vi "Execute Commands.vi"(8 "error in (no error)":errorcluster, 10 "Command Array":refnum<class "Command.lvclass">[](array[class]), 11 "Command Handler in":refnum<class "Command Handler.lvclass">) -> (0 "error out":errorcluster, 3 "Command Handler out":refnum<class "Command Handler.lvclass">)   [LabVIEW 2015, in "Command Handler.lvlib" / "Command Handler.lvclass"]
uses:
  Command Handler.lvclass
  Command Handler Messages/Command Handler Global API/Command Handler Global.vi
  Command Handler.lvlib
  Command Parent/Command.lvclass
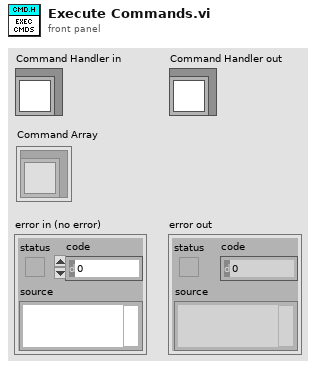
[diagram p1: front panel]
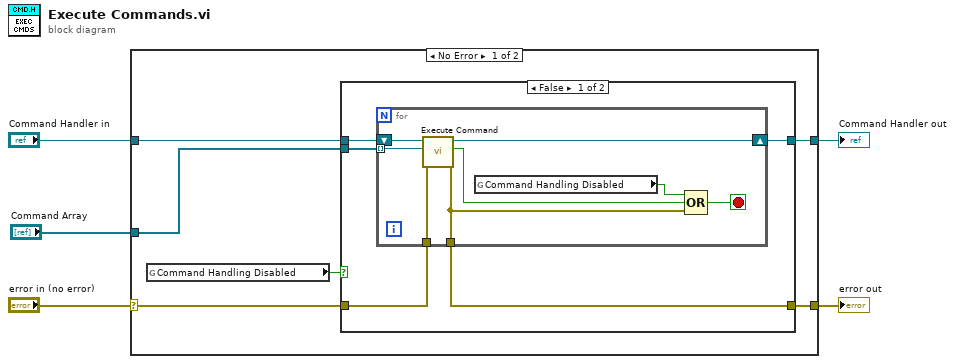
[diagram p0: block diagram]
diagram:
  n1 = case shown="No Error" "error in (no error)" {
    selector: "error in (no error)" -> [w10 w28]
    tunnel: [w9 w28] -> w4
    tunnel: [w7 w27] -> w2
    tunnel: "Command Handler in" -> [w8 w27]
    tunnel: "Command Array" -> [w11 _]
    frame No Error {
      n2 = global read "Command Handler Global.vi" "Command Handling Disabled"() -> (w6:bool)
      n3 = case shown="False" w6 {
        tunnel: w11 -> [w16 _]
        tunnel: w10 -> [w15 w25]
        tunnel: [w14 w25] -> w9
        tunnel: w8 -> [w13 w26]
        tunnel: [w12 w26] -> w7
        frame False {
          n4 = for {
            tunnel: w16 -> [w21] mode=indexing
            tunnel: w15 -> [w22]
            tunnel: [w19] -> w14
            shift-right: [w23] -> w12
            shift-left: w13 -> [w24]
            stop <- w18 stop-if-true
            n5 = call-dynamic "Execute Command.vi"("error in (no error)"=w22, "Command"=w21, "Command Handler in"=w24) -> ("error out"=w19:errorcluster, "Stop"=w20:bool, "Command Handler out"=w23:refnum<class "Command Handler.lvclass">)  [unwired: 6 in]
            n6 = global read "Command Handler Global.vi" "Command Handling Disabled"() -> (w17:bool)
            n7 = Compound Arithmetic op=OR(w17, w20, w19) -> (w18:bool)
          }
        }
        frame True {
        }
      }
    }
    frame Error {
    }
  }
  "error out" <- w4
  "Command Handler out" <- w2
